vi "Draw circles .vi"(1 "Circles":cluster{"x":dbl, "y":dbl, "r":dbl}[](array[cluster]), 2 "Refnum in":T1) -> (0 "Refnum out":T1)   [LabVIEW 2018]
uses:
  <vilib>/vision/Image Controls.llb/IMAQ Image.ctl
  vision info 2.vi
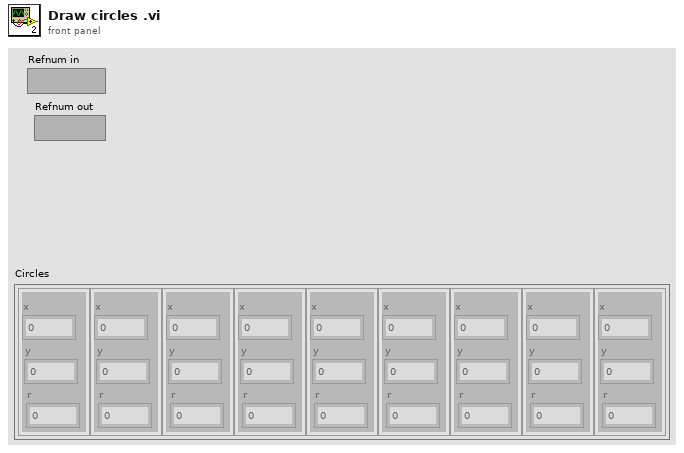
[diagram p1: front panel]
types:
  T1 = typedef "IMAQ Image.ctl" = refnum<image>
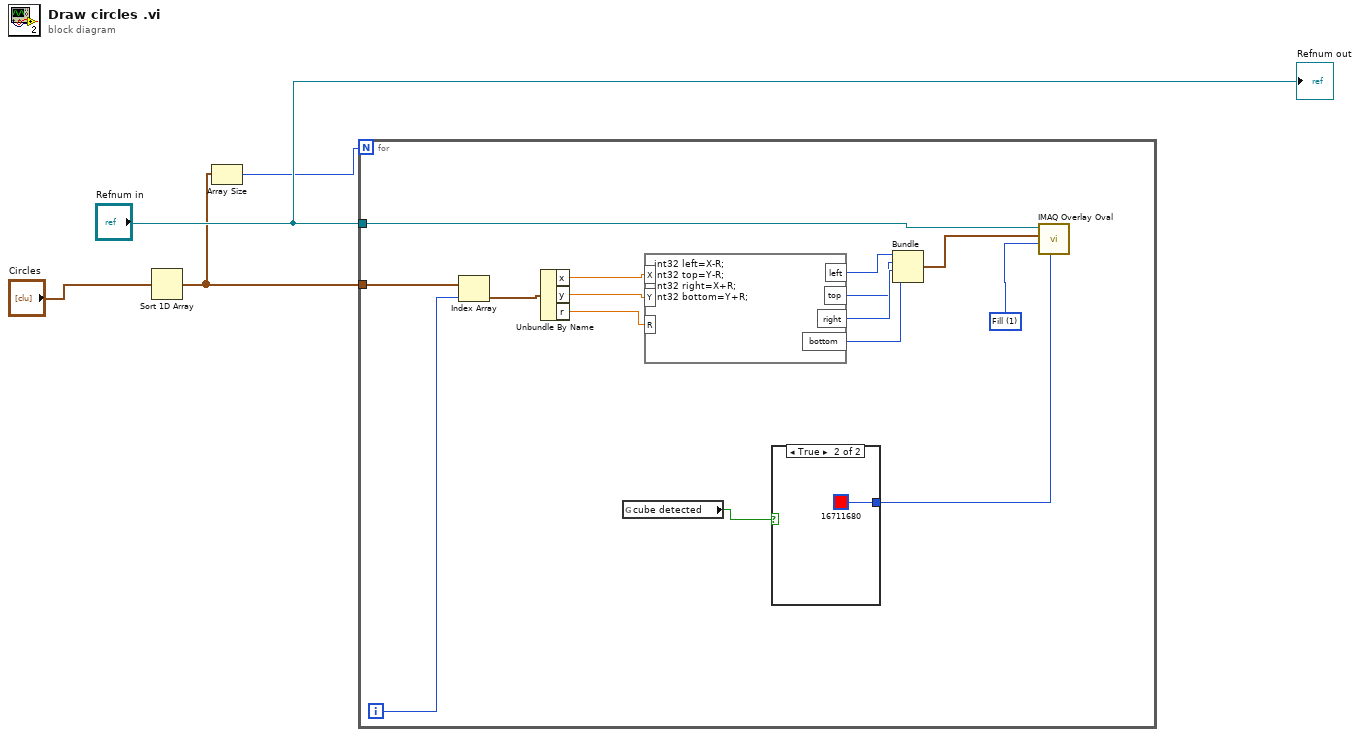
[diagram p0: block diagram]
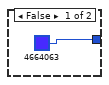
[diagram p2: hidden frame]
diagram:
  n1 = Sort 1D Array(array="Circles") -> (sorted array=w2:cluster{"x":dbl, "y":dbl, "r":dbl}[])
  n2 = Array Size(array=w2) -> (size(s)=w3:i32)
  n3 = for {
    N: w3 -> [_]
    tunnel: w2 -> [w13]
    tunnel: "Refnum in" -> [w12]
    i -> [w11]
    w19 = u32 1 items=["Frame", "Fill"] ("Drawing Mode (Frame)")
    n4 = Index Array(array=w13, index=w11) -> (element=w10:cluster{"x":dbl, "y":dbl, "r":dbl})
    n5 = Unbundle By Name(w10) -> ("x"=w7:dbl, "y"=w8:dbl, "r"=w9:dbl)
    n6 = global read "vision info 2.vi" "cube detected"() -> (w5:bool)
    n7 = formula code="int32 left=X-R;\nint32 top=Y-R;\nint32 right=X+R;\nint32 bottom=Y+R;"("X"=w7, "Y"=w8, "R"=w9) -> ("left"=w14:i32, "top"=w15:i32, "right"=w16:i32, "bottom"=w17:i32)
    n8 = case shown="True" w5 {
      tunnel: [u32 4664063 ("Color") u32 16711680 ("Color")] -> w6
      frame False {
      }
      frame True {
      }
    }
    n9 = Bundle(w14, w15, w16, w17) -> (w18:cluster{i32, i32, i32, i32})  [unwired: 1 in]
    n10 = call "IMAQ Overlay Oval"("Color"=w6, "Drawing Mode (Frame)"=w19, "Bounding Rectangle"=w18, "Image"=w12) -> ()  [unwired: 6 in, 2 out]
  }
  "Refnum out" <- "Refnum in"
